vi "aft_xmpl_QAM (PtbyPt).vi"() -> (3 "QAM signal":cdb)   [LabVIEW 2023]
uses:
  <vilib>/ptbypt/NI_PtbyPt.lvlib
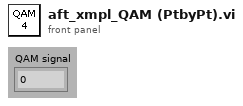
[diagram p1: front panel]
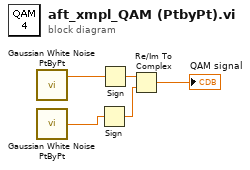
[diagram p0: block diagram]
diagram:
  n1 = call <vilib>:"Gaussian White Noise PtByPt.vi"() -> ("Gaussian white noise"=w3:dbl)  [unwired: 3 in]
  n2 = call <vilib>:"Gaussian White Noise PtByPt.vi"() -> ("Gaussian white noise"=w5:dbl)  [unwired: 3 in]
  n3 = Sign(1:w5) -> (0:w4:dbl)
  n4 = Sign(1:w3) -> (0:w2:dbl)
  n5 = Re/Im To Complex(1:w4, 2:w2) -> (0:→"QAM signal":cdb)
